vi "PythonConverter_GUI.vi"(5 "Build Directory":path, 6 "error in":errorcluster, 9 "VI Interpreter":refnum<class "VI Interpreter.lvclass">) -> (0 "error out":errorcluster, 3 "PythonConverter_GUI out":refnum<class "PythonConverter_GUI.lvclass">)   [LabVIEW 2014, in "Raspberry Pi Compatible Compiler for LabVIEW.lvlib" / "PythonConverter_GUI.lvclass"]
uses:
  PythonConverter_GUI.lvclass
  VI Interpreter/Classes/VI Interpreter/VI Interpreter.lvclass
  PythonConverter_GUI.lvclass/PythonConverter_GUI.ctl
  PythonConfiguration/PythonConfiguration.lvclass
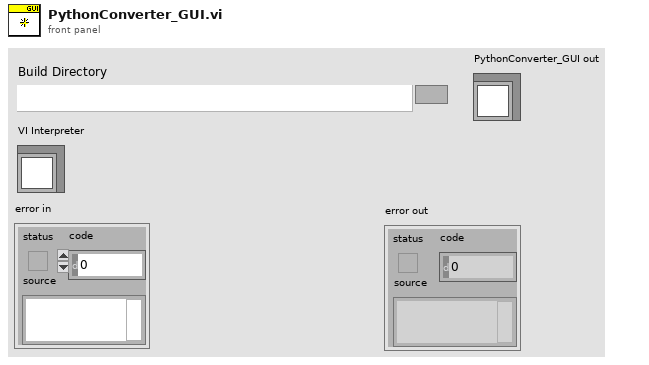
[diagram p1: front panel]
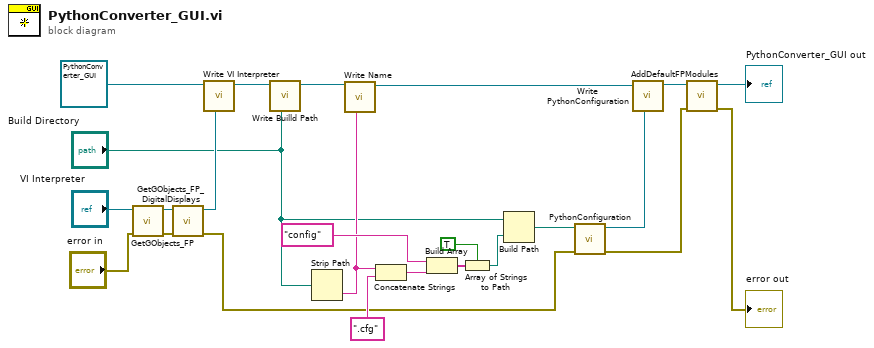
[diagram p0: block diagram]
diagram:
  n1 = call "GetGObjects_FP.vi"("error in"="error in", "VI Interpreter in"="VI Interpreter") -> ("error out"=w7:errorcluster, "VI Interpreter out"=w6:refnum<class "VI Interpreter.lvclass">)  [unwired: 8 in]
  n2 = call "GetGObjects_FP_DigitalDisplays.vi"("error in"=w7, "VI Interpreter in"=w6) -> ("error out"=w1:errorcluster, "VI Interpreter out"=w5:refnum<class "VI Interpreter.lvclass">)  [unwired: 8 in]
  n3 = call "Write VI Interpreter.vi"("VI Interpreter"=w5, "PythonConverter_GUI in"=refnum<class "PythonConverter_GUI.lvclass"> refnum) -> ("PythonConverter_GUI out"=w8:refnum<class "PythonConverter_GUI.lvclass">)  [unwired: 7 in]
  n4 = call "Write Builld Path.vi"("Builld Path"="Build Directory", "PythonConverter_GUI in"=w8) -> ("PythonConverter_GUI out"=w16:refnum<class "PythonConverter_GUI.lvclass">)  [unwired: 7 in]
  n5 = Strip Path(path="Build Directory") -> (name=w22:string)  [unwired: 1 out]
  n6 = call "Write Name.vi"("Name"=w22, "PythonConverter_GUI in"=w16) -> ("PythonConverter_GUI out"=w15:refnum<class "PythonConverter_GUI.lvclass">)  [unwired: 7 in]
  n7 = Concatenate Strings(w22, ".cfg" ("string")) -> (w23:string)
  n8 = Build Array("config" ("name or relative path"), w23) -> (w20:string[])
  n9 = Array of Strings to Path(0:w20, 1:TRUE ("relative")) -> (2:w18:path)
  n10 = Build Path(base path="Build Directory", name or relative path=w18) -> (appended path=w17:path)
  n11 = call "PythonConfiguration.vi"("error in"=w1, "Configuration Path"=w17) -> ("error out"=w11:errorcluster, "PythonConfiguration out"=w14:refnum<class "PythonConfiguration.lvclass">)  [unwired: 8 in]
  n12 = call "Write PythonConfiguration.vi"("PythonConfiguration"=w14, "PythonConverter_GUI in"=w15) -> ("PythonConverter_GUI out"=w13:refnum<class "PythonConverter_GUI.lvclass">)  [unwired: 7 in]
  n13 = call "AddDefaultFPModules.vi"("error in"=w11, "PythonConverter_GUI in"=w13) -> ("error out"=→"error out":errorcluster, "PythonConverter_GUI out"=→"PythonConverter_GUI out":refnum<class "PythonConverter_GUI.lvclass">)  [unwired: 6 in]
